vi "Update Decay & IRF Parameters.vi"(8 "Error In":errorcluster, 11 "Decay & IRF Parameters Refnum":refnum<vi>) -> (0 "error out":errorcluster, 1 "Value":T1 {"Lifetime" min=0.0; "IRF Period" min=0.0}, 2 "Laser Period":dbl[unit], 3 "Decay & IRF Parameters Refnum":refnum<vi>)   [LabVIEW 2019]
uses:
  Phasor Explorer Decay Parameters.ctl
  IRF Model.ctl
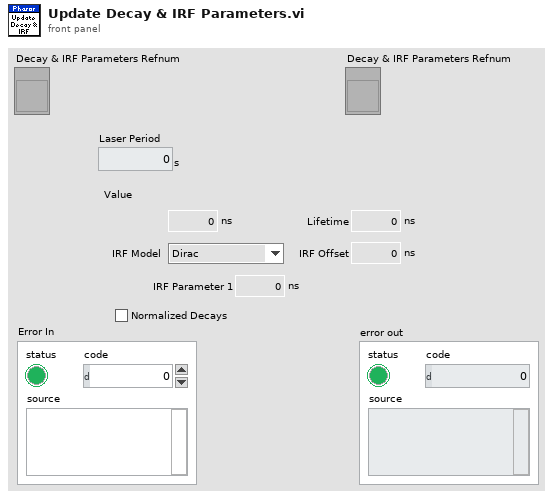
[diagram p1: front panel]
types:
  T1 = typedef "Phasor Explorer Decay Parameters.ctl" = cluster{"Lifetime":dbl[unit], "IRF Offset":dbl[unit], "IRF Period":dbl[unit], "Normalized Decays":bool, "IRF Model":T2, "IRF Parameter 1":dbl[unit]}
  T2 = typedef "IRF Model.ctl" = enum16{"Dirac", "Exponential"}
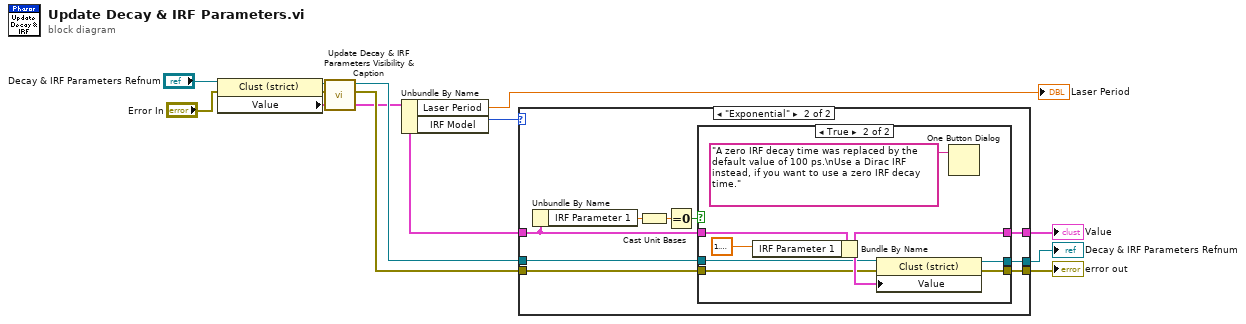
[diagram p0: block diagram]
diagram:
  n1 = property class="Clust (strict)"(reference="Decay & IRF Parameters Refnum", error in="Error In") -> (reference out=w7:refnum<vi>, error out=w11:errorcluster, "Value"=w5:T1)
  n2 = call "Update Decay & IRF Parameters Visibility & Caption.vi"("error in (no error)"=w11, "Phasor Explorer Decay & IRF Parameters in"=w7) -> ("error out"=w12:errorcluster, "Phasor Explorer Decay & IRF Parameters out"=w10:refnum<vi>)  [unwired: 8 in]
  n3 = Unbundle By Name(w5) -> ("Laser Period"=→"Laser Period":dbl[unit], "IRF Model"=w4:T2)
  n4 = case shown="\"Exponential\"" w4 {
    tunnel: w5 -> [w15 w21]
    tunnel: [w15 w20] -> w6
    tunnel: w10 -> [w14 w19]
    tunnel: [w14 w18] -> w8
    tunnel: w12 -> [w13 w17]
    tunnel: [w13 w16] -> w9
    frame "Dirac", Default {
    }
    frame "Exponential" {
      n5 = Unbundle By Name(w21) -> ("IRF Parameter 1"=w24:dbl[unit])
      n6 = Cast Unit Bases(0:w24) -> (2:w23:dbl)  [unwired: 1 in]
      n7 = Equal To 0?(x=w23) -> (x = 0?=w22:bool)
      n8 = case shown="True" w22 {
        tunnel: w21 -> [w27 w34]
        tunnel: [w27 w32] -> w20
        tunnel: w19 -> [w26 w31]
        tunnel: [w26 w30] -> w18
        tunnel: w17 -> [w25 w29]
        tunnel: [w25 w28] -> w16
        frame False {
        }
        frame True {
          n9 = Bundle By Name(cluster=w34, "IRF Parameter 1"=dbl[unit] 1.0000000000000002e-10) -> (w32:T1)
          n10 = property class="Clust (strict)"(reference=w31, error in=w29, "Value"=w32) -> (reference out=w30:refnum<vi>, error out=w28:errorcluster)
          n11 = One Button Dialog(message="A zero IRF decay time was replaced by the default value of 100 ps.\nUse a Dirac IRF instead, if you want to use a zero IRF decay time.") -> ()  [unwired: 1 in, 1 out]
        }
      }
    }
  }
  "error out" <- w9
  "Decay & IRF Parameters Refnum" <- w8
  "Value" <- w6
